vi "Network Steam Read Message.vi"(6 "Timeout(ms)":i32, 8 "error in (no error)":errorcluster, 11 "Model_AMC in":refnum<class "Model_AMC.lvclass">) -> (0 "error out":errorcluster, 1 "Message":T1, 2 "StillConnected?":bool, 3 "Model_AMC out":refnum<class "Model_AMC.lvclass">, 4 "Timed Out?":bool)   [LabVIEW 2021, in "Model_AMC.lvclass"]
uses:
  Model_AMC.lvclass
  Model_AMC.lvclass/Model_AMC.ctl
  <userlib>/John_Lib/Network_Streams_Connection/NetworkConnection.lvclass
  <userlib>/John_Lib/Network_Streams_Connection/NetworkCommand--Cluster.ctl
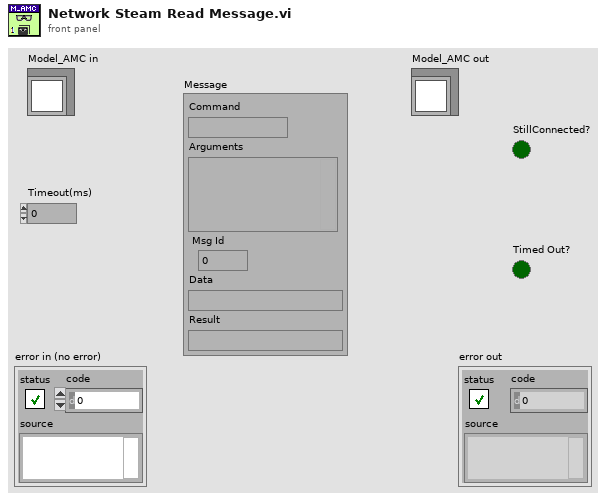
[diagram p1: front panel]
types:
  T1 = typedef "JKI_Network_Streams.lvlib/NetworkConnection.lvclass/NetworkCommand--Cluster.ctl" = cluster{"Command":string, "Arguments":variant, " Msg Id":i32, "Data":string, "Result":string}
  T2 = typedef "Model_AMC.lvclass/DVR.ctl" = cluster{"JKI_Network_Streams":refnum<class "NetworkConnection.lvclass">, "AMC Q":T3, "Connnected":bool}
  T3 = typedef "Model_AMC.lvclass/AMC Q.ctl" = cluster{"Main":T4, "OPCUA":T4, "NetworkSteam":T4}
  T4 = typedef "AMC_FW.lvlib/Queue.ctl" = cluster{"Q":T5, "Name":string}
  T5 = typedef "AMC_FW.lvlib/Message Queue.ctl" = refnum<queue>
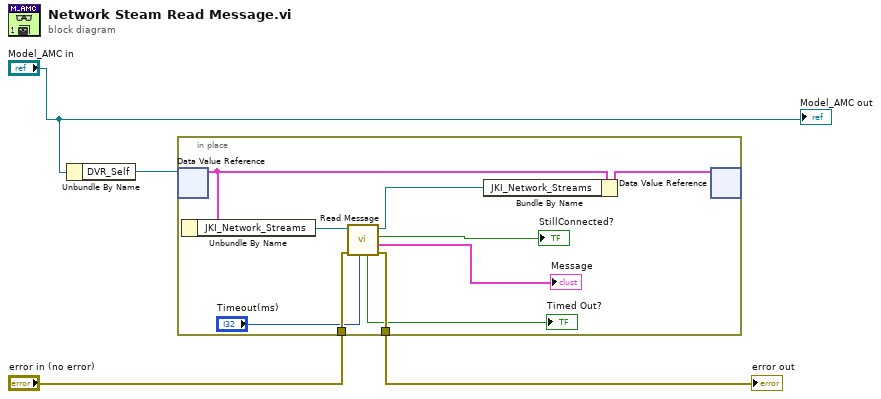
[diagram p0: block diagram]
diagram:
  n1 = Unbundle By Name("Model_AMC in") -> ("DVR_Self"=w4:refnum<data-value>)
  n2 = in-place {
    in-place-border: "error in (no error)" -> [w10]
    in-place-border: [w8] -> w2
    n3 = in-place-dvr #1(w4) -> (w14:T2)  [unwired: 1 out]
    n4 = Unbundle By Name(w14) -> ("JKI_Network_Streams"=w13:refnum<class "NetworkConnection.lvclass">)
    n5 = call <userlib>:"Read Message.vi"("Timeout(ms)"="Timeout(ms)", "error in (no error)"=w10, "NetworkConnection in"=w13) -> ("error out"=w8:errorcluster, "Message"=→"Message":T1, "StillConnected?"=→"StillConnected?":bool, "NetworkConnection out"=w11:refnum<class "NetworkConnection.lvclass">, "Timed Out?"=→"Timed Out?":bool)  [unwired: 3 in, 1 out]
    n6 = Bundle By Name(cluster=w14, "JKI_Network_Streams"=w11) -> (w12:T2)
    n7 = in-place-dvr #1(w12) -> ()  [unwired: 2 out]
  }
  "error out" <- w2
  "Model_AMC out" <- "Model_AMC in"
